vi "Verdichternamen.vi"(11 "Array":dbl[](array[numeric])) -> (3 "Dynamic Data":dynamicdata(waveform))   [LabVIEW 2015]
uses:
  <vilib>/express/express shared/transition.llb/Dynamic To Waveform Array.vi
  <vilib>/express/express signal manip/GetorSetDDTAttributes/Set DDT Attributes/SetT0.vi
  <vilib>/express/express shared/transition.llb/Waveform Array To Dynamic.vi
  <vilib>/express/express signal manip/GetorSetDDTAttributes/Set DDT Attributes/Set DDT Properties.xnode
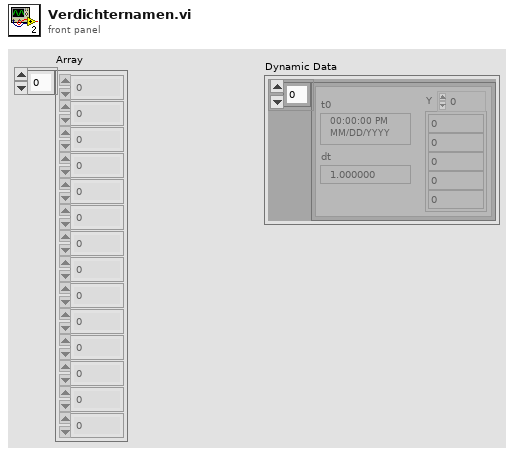
[diagram p1: front panel]
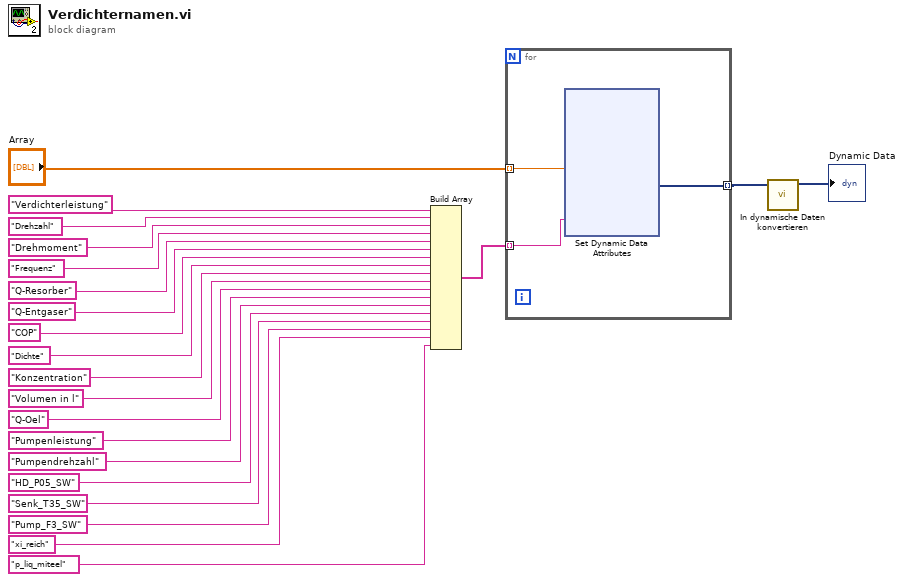
[diagram p0: block diagram]
diagram:
  n1 = Build Array("Verdichterleistung", "Drehzahl", "Drehmoment", "Frequenz", "Q-Resorber", "Q-Entgaser", "COP", "Dichte", "Konzentration", "Volumen in l", "Q-Oel", "Pumpenleistung", "Pumpendrehzahl", "HD_P05_SW", "Senk_T35_SW", "Pump_F3_SW", "xi_reich", "p_liq_miteel") -> (w21:string[])
  n2 = for {
    tunnel: "Array" -> [w25] mode=indexing
    tunnel: w21 -> [w24] mode=indexing
    tunnel: [w23] -> w13 mode=indexing
    n3 = xnode "Set Dynamic Data Attributes"("Signals In"=w25, "Signal Name"=w24) -> ("Signals Out"=w23:dynamicdata)  [unwired: 2 in, 1 out]
  }
  n4 = call "In dynamische Daten konvertieren"("Array of Waveforms"=w13) -> ("Dynamic Data Type"=→"Dynamic Data":dynamicdata)  [unwired: 3 in]
